vi "NewEraPump Stop Pumps Edited.vi"(2 "error in (no error)":errorcluster, 3 "VISA resource name":refnum<visa-resource-name>="COM1", 4 "Secondary Pump Address (0)":i32 format="%0#.0f", 5 "Master Pump Address (0)":i32 format="%0#.0f") -> (0 "error out":errorcluster, 1 "VISA resource name out":refnum<visa-resource-name>)   [LabVIEW 2020]
doc: "Stop/pauses the pumping program."
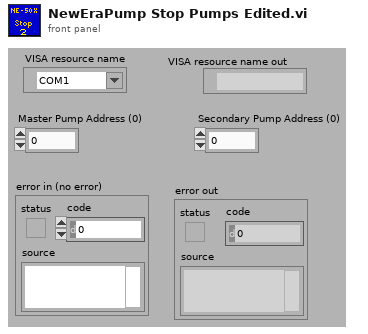
[diagram p1: front panel]
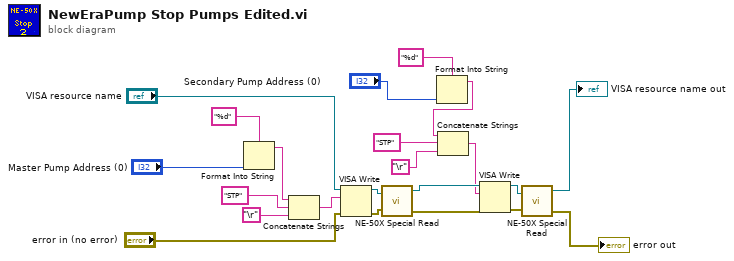
[diagram p0: block diagram]
diagram:
  n1 = Format Into String(format string="%d", "Master Pump Address (0)") -> (resulting string=w13:string)  [unwired: 2 in, 1 out]
  n2 = Concatenate Strings(w13, "STP", "\r") -> (w19:string)
  n3 = VISA Write(VISA resource name="VISA resource name", write buffer=w19, error in (no error)="error in (no error)") -> (VISA resource name out=w16:refnum<visa-resource-name>, error out=w17:errorcluster)  [unwired: 1 out]
  n4 = call <instrlib>:"NE-50X Special Read.vi"("VISA resource name"=w16, "error in (no error)"=w17) -> ("VISA resource name out"=w8:refnum<visa-resource-name>, "error out"=w7:errorcluster)  [unwired: 1 out]
  n5 = Format Into String(format string="%d", "Secondary Pump Address (0)") -> (resulting string=w4:string)  [unwired: 2 in, 1 out]
  n6 = Concatenate Strings(w4, "STP", "\r") -> (w1:string)
  n7 = VISA Write(VISA resource name=w8, write buffer=w1, error in (no error)=w7) -> (VISA resource name out=w12:refnum<visa-resource-name>, error out=w11:errorcluster)  [unwired: 1 out]
  n8 = call <instrlib>:"NE-50X Special Read.vi"("VISA resource name"=w12, "error in (no error)"=w11) -> ("VISA resource name out"=→"VISA resource name out":refnum<visa-resource-name>, "error out"=→"error out":errorcluster)  [unwired: 1 out]
